vi "发送报表至邮箱.vi"() -> ()   [LabVIEW 2009]
panel:
  in  "邮件内容":string="设备运行状态"
  in  "发送目的邮箱":string
  in  "邮件主题":string="故障诊断"
  in  "发送邮件的附件":path
  in  "密码":string
  in  "邮箱发送服务器":string="smtp.163.com"
  in  "您的邮箱名":string
  out "error out":errorcluster
  # "您的用来发送的邮箱的密码！"
  # "您的邮箱登陆名"
  # "邮箱发送服务器的地址"
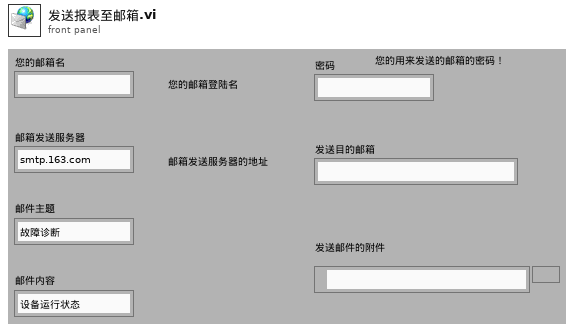
[diagram p1: front panel]
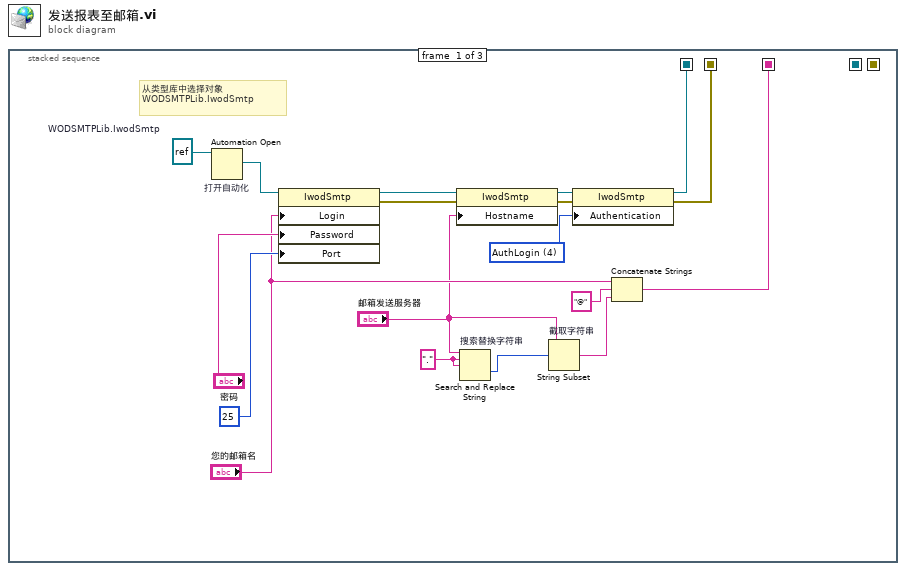
[diagram p0: block diagram]
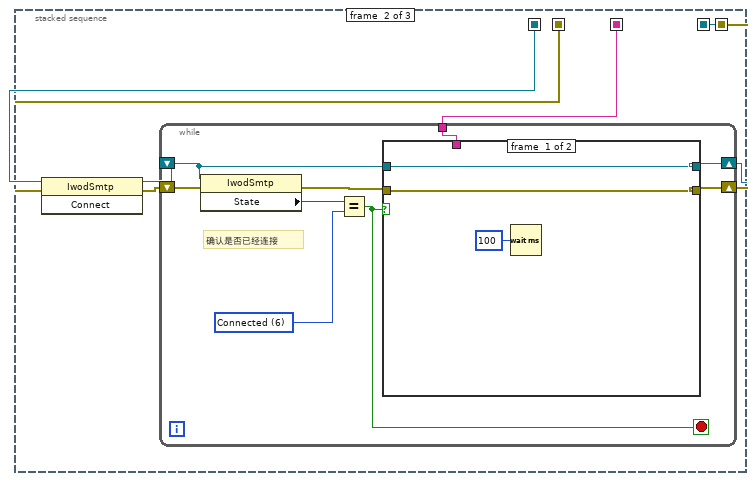
[diagram p2: hidden frame]
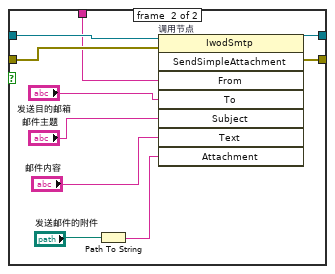
[diagram p3: hidden frame]
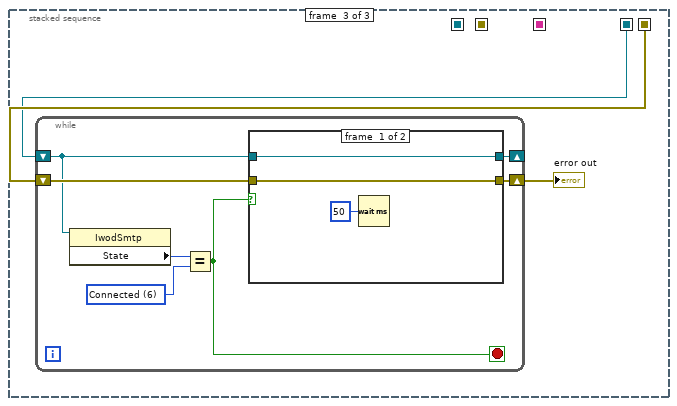
[diagram p4: hidden frame]
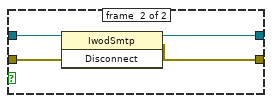
[diagram p5: hidden frame]
diagram:
  n1 = stacked-sequence {
    seq-local: [w11 _ _] -> [_ w25 _]
    seq-local: [w10 _ _] -> [_ w24 _]
    seq-local: [_ w20 _] -> [_ _ w48]
    seq-local: [_ w22 _] -> [_ _ w50]
    seq-local: [w7 _ _] -> [_ w19 _]
    frame #0 {
      w3 = refnum<k7> refnum  # WODSMTPLib.IwodSmtp
      w9 = "." ("search string")
      w18 = 4 items=["AuthNone"=1, "AuthLogin"=4, "AuthPlain"=8, "AuthCramMD5"=16] ("Authentication")
      # "从类型库中选择对象\nWODSMTPLib.IwodSmtp"
      n2 = Automation Open "打开自动化"(Automation Refnum=w3) -> (Automation Refnum=w2:refnum<k7>)  [unwired: 3 in, 1 out]
      n3 = property class="IwodSmtp"(reference=w2, "Login"="您的邮箱名", "Password"="密码", "Port"=25) -> (reference out=w14:refnum<k7>, error out=w17:errorcluster)  [unwired: 1 in]
      n4 = property class="IwodSmtp"(reference=w14, error in=w17, "Hostname"="邮箱发送服务器") -> (reference out=w15:refnum<k7>, error out=w16:errorcluster)
      n5 = Search and Replace String "搜索替换字符串"(input string="邮箱发送服务器", search string=w9, replace string=w9) -> (offset past replacement=w6:i32)  [unwired: 5 in, 3 out]
      n6 = String Subset "截取字符串"(string="邮箱发送服务器", offset (0)=w6) -> (substring=w5:string)  [unwired: 1 in]
      n7 = property class="IwodSmtp"(reference=w15, error in=w16, "Authentication"=w18) -> (reference out=w11:refnum<k7>, error out=w10:errorcluster)
      n8 = Concatenate Strings("您的邮箱名", "@" ("string"), w5) -> (w7:string)
    }
    frame #1 {
      n9 = invoke class="IwodSmtp" method="Connect"(reference=w25, error in=w24) -> (reference out=w21:refnum<k7>, error out=w23:errorcluster)  [unwired: 1 in, 1 out]
      n10 = while {
        shift-right: [w31] -> w22
        shift-left: w23 -> [w33]
        shift-right: [w29] -> w20
        shift-left: w21 -> [w30]
        tunnel: w19 -> [w28]
        stop <- w34 stop-if-true
        w27 = 6 items=["Disconnected", "RelayResolvingMX", "RelayResolvingA", "Connecting", "SendingGreeting", "LogonInProgress", "Connected", "SendingMailFrom", "SendingRcptTo", "SendingData", "SendingHeaders", "SendingBody", "Resetting", "Completed", "Retrying", "NegotiatingSSL", "EstablishedSSL"] ("State")
        # "确认是否已经连接"
        n11 = property class="IwodSmtp"(reference=w30, error in=w33) -> (error out=w32:errorcluster, "State"=w26:i32)  [unwired: 1 out]
        n12 = Equal?(x=w26, y=w27) -> (x = y?=w34:bool)
        n13 = case shown="真" w34 {
          tunnel: w30 -> [w37 w47]
          tunnel: [w37 w46] -> w29
          tunnel: w32 -> [w36 w45]
          tunnel: [w36 w44] -> w31
          tunnel: w28 -> [_ w43]
          frame #0 {
            n14 = Wait (ms)(milliseconds to wait=u32 100) -> ()  [unwired: 1 out]
          }
          frame #1 {
            n15 = Path To String(path="发送邮件的附件") -> (string=w39:string)
            n16 = invoke on="调用节点" class="IwodSmtp" method="SendSimpleAttachment"(reference=w47, error in=w45, "From"=w43, "To"="发送目的邮箱", "Subject"="邮件主题", "Text"="邮件内容", "Attachment"=w39) -> (reference out=w46:refnum<k7>, error out=w44:errorcluster)  [unwired: 1 in, 6 out]
          }
        }
      }
    }
    frame #2 {
      n17 = while {
        shift-right: [w57] -> w49
        shift-left: w50 -> [w55]
        shift-right: [w56] -> _
        shift-left: w48 -> [w54]
        stop <- w52 stop-if-true
        w53 = 6 items=["Disconnected", "RelayResolvingMX", "RelayResolvingA", "Connecting", "SendingGreeting", "LogonInProgress", "Connected", "SendingMailFrom", "SendingRcptTo", "SendingData", "SendingHeaders", "SendingBody", "Resetting", "Completed", "Retrying", "NegotiatingSSL", "EstablishedSSL"] ("State")
        n18 = property class="IwodSmtp"(reference=w54) -> ("State"=w51:i32)  [unwired: 1 in, 2 out]
        n19 = Equal?(x=w51, y=w53) -> (x = y?=w52:bool)
        n20 = case shown="真" w52 {
          tunnel: w54 -> [w60 w64]
          tunnel: [w60 w61] -> w56
          tunnel: w55 -> [w59 w63]
          tunnel: [w59 w62] -> w57
          frame #0 {
            n21 = Wait (ms)(milliseconds to wait=u32 50) -> ()  [unwired: 1 out]
          }
          frame #1 {
            n22 = invoke class="IwodSmtp" method="Disconnect"(reference=w64, error in=w63) -> (reference out=w61:refnum<k7>, error out=w62:errorcluster)  [unwired: 1 in, 1 out]
          }
        }
      }
      "error out" <- w49
    }
  }
